vi "GenerateTriggeredStimulus.vi"(8 "error in (no error)":errorcluster, 11 "Stimulus in":refnum<class "HeadandTailRailswithDelay.lvclass">) -> (0 "error out":errorcluster, 2 "TriggeredStimulus":sgl[][](array[numeric]), 3 "Stimulus out":refnum<class "HeadandTailRailswithDelay.lvclass">)   [LabVIEW 2019, in "HeadandTailRailswithDelay.lvclass"]
uses:
  HeadandTailRailswithDelay.lvclass
  HeadandTailRailswithDelay.lvclass/HeadandTailRailswithDelay.ctl
  ParametersGlobal.vi
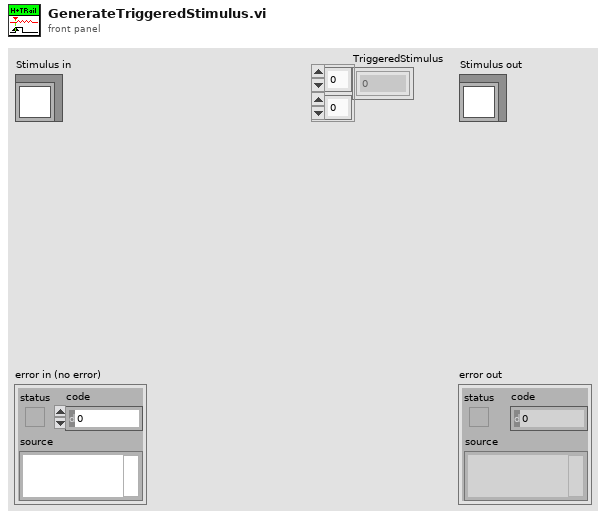
[diagram p1: front panel]
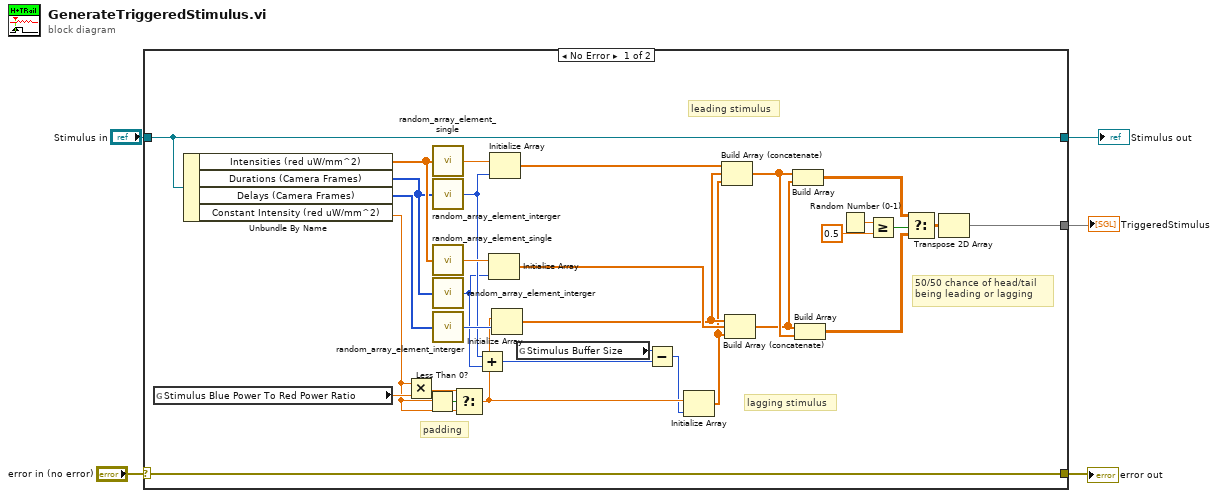
[diagram p0: block diagram]
diagram:
  n1 = case shown="No Error" "error in (no error)" {
    selector: "error in (no error)" -> [w19 w38]
    tunnel: [w19 w38] -> w2
    tunnel: [w31 w37] -> w4
    tunnel: "Stimulus in" -> [w31 w37]
    tunnel: [w35 _] -> w3
    frame No Error {
      # "padding"
      # "lagging stimulus"
      # "leading stimulus"
      # "50/50 chance of head/tail \nbeing leading or lagging"
      n2 = global read "ParametersGlobal.vi" "Stimulus Blue Power To Red Power Ratio"() -> (w32:sgl)
      n3 = Unbundle By Name(w31) -> ("Intensities (red uW/mm^2)"=w23:sgl[], "Durations (Camera Frames)"=w22:i32[], "Delays (Camera Frames)"=w21:i32[], "Constant Intensity (red uW/mm^2)"=w30:sgl)
      n4 = Multiply(x=w30, y=w32) -> (x*y=w34:sgl)
      n5 = Less Than 0?(x=w30) -> (x < 0?=w33:bool)
      n6 = call "random_array_element_single.vi"("Array of numbers"=w23) -> ("Randomly selected number"=w36:sgl)
      n7 = call "random_array_element_interger.vi"("Array of numbers"=w22) -> ("Randomly selected number"=w8:i32)
      n8 = call "random_array_element_single.vi"("Array of numbers"=w23) -> ("Randomly selected number"=w20:sgl)
      n9 = call "random_array_element_interger.vi"("Array of numbers"=w22) -> ("Randomly selected number"=w7:i32)
      n10 = call "random_array_element_interger.vi"("Array of numbers"=w21) -> ("Randomly selected number"=w18:i32)
      n11 = Select(t=w34, s=w33, f=w30) -> (s? t:f=w13:sgl)
      n12 = Add(x=w8, y=w7) -> (x+y=w9:i32)
      n13 = Initialize Array(w20, w7) -> (w17:sgl[])
      n14 = Initialize Array(w36, w8) -> (w16:sgl[])
      n15 = Initialize Array(w13, w18) -> (w15:sgl[])
      n16 = global read "ParametersGlobal.vi" "Stimulus Buffer Size"() -> (w11:i32)
      n17 = Subtract(x=w11, y=w9) -> (x-y=w10:i32)
      n18 = Initialize Array(w13, w10) -> (w6:sgl[])
      n19 = Build Array (concatenate)(w16, w15, w6) -> (w14:sgl[])
      n20 = Build Array (concatenate)(w15, w17, w6) -> (w12:sgl[])
      n21 = Build Array(w14, w12) -> (w26:sgl[][])
      n22 = Build Array(w12, w14) -> (w25:sgl[][])
      n23 = Random Number (0-1)() -> (number: 0 to 1=w29:dbl)
      n24 = Greater Or Equal?(x=w29, y=0.5) -> (x >= y?=w27:bool)
      n25 = Select(t=w26, s=w27, f=w25) -> (s? t:f=w24:sgl[][])
      n26 = Transpose 2D Array(2D array=w24) -> (transposed array=w35:sgl[][])
    }
    frame Error {
    }
  }
  "error out" <- w2
  "Stimulus out" <- w4
  "TriggeredStimulus" <- w3
